vi "implementation error.vi"(8 "error in (no error)":errorcluster, 11 "params":variant) -> (0 "error out":errorcluster, 3 "data":variant)   [LabVIEW 2017]
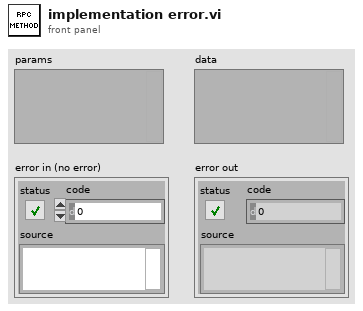
[diagram p1: front panel]
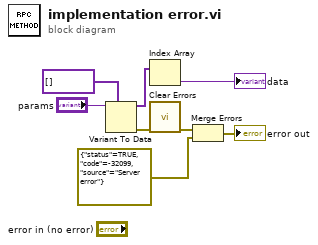
[diagram p0: block diagram]
diagram:
  n1 = Variant To Data(type=variant[] [], Variant="params") -> (data=w5:variant[], error out=w4:errorcluster)  [unwired: 1 in]
  n2 = Index Array(array=w5) -> (element=→"data":variant)  [unwired: 1 in]
  n3 = call <vilib>:"Clear Errors.vi"("error in (no error)"=w4) -> ("error out"=w1:errorcluster)  [unwired: 5 in, 1 out]
  n4 = Merge Errors(w1, errorcluster {"status"=TRUE, "code"=-32099, "source"="Server error"} ("error out")) -> (→"error out":errorcluster)
